vi "UI_Example.vi"() -> ()   [LabVIEW 2018]
uses:
  UI_Library/UI_Library.lvclass
  test/ClassData/ClassData.lvclass
  UI_Library.lvlib
  d44c3c8a-f4a9-44f0-87a1-e82cc9f3e378.vi
  bafeb2e0-969a-4f59-9125-878fceaa8550.vi
panel:
  in  "UI_Cluster":cluster{"Strg":string}
  out "Stopped":bool
  in  "Stop":bool
  out "NewVal":bool
  in  "UI_Strg":string
  in  "UI_Boolean":bool
  out "#el_queue":i32
  # "Example\nThis example highlights how the new library enables a fully decoupled architecture, allowing the Backend logic to operate independently and effortlessly from the UI layer.\nThanks to this library, UI interaction becomes cleaner, safer, and dramatically easier to maintain.\nSee Block Diagram Comment for more details!\n\nAnd the best part:\nThe library automatically manages all UI control references—zero boilerplate, zero coupling, maximum flexibility\nThe UI stays continuously updated by reference using a dedicated loop, ensuring smooth UI responsiveness without ever slowing down the Backend"
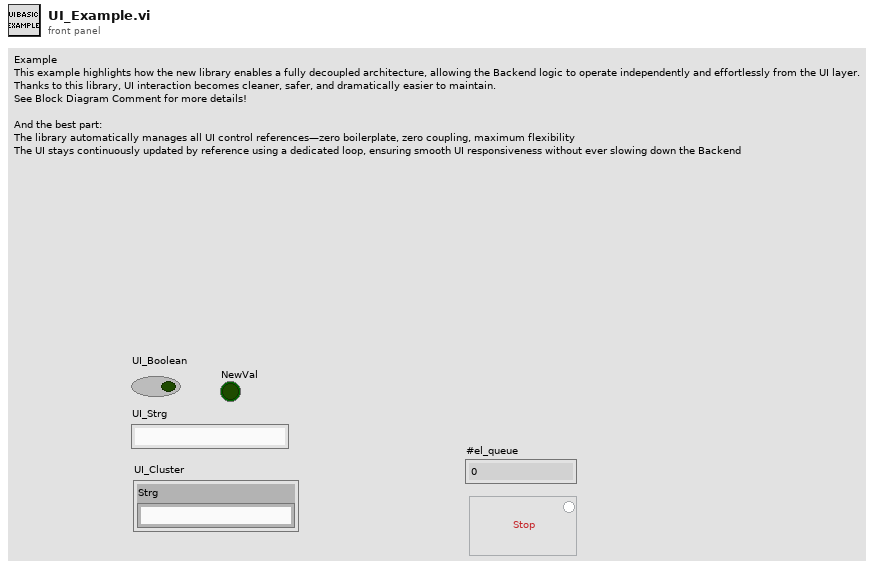
[diagram p1: front panel]
types:
  T1 = enum8{"Enabled", "Disabled", "Disabled and Grayed Out"}
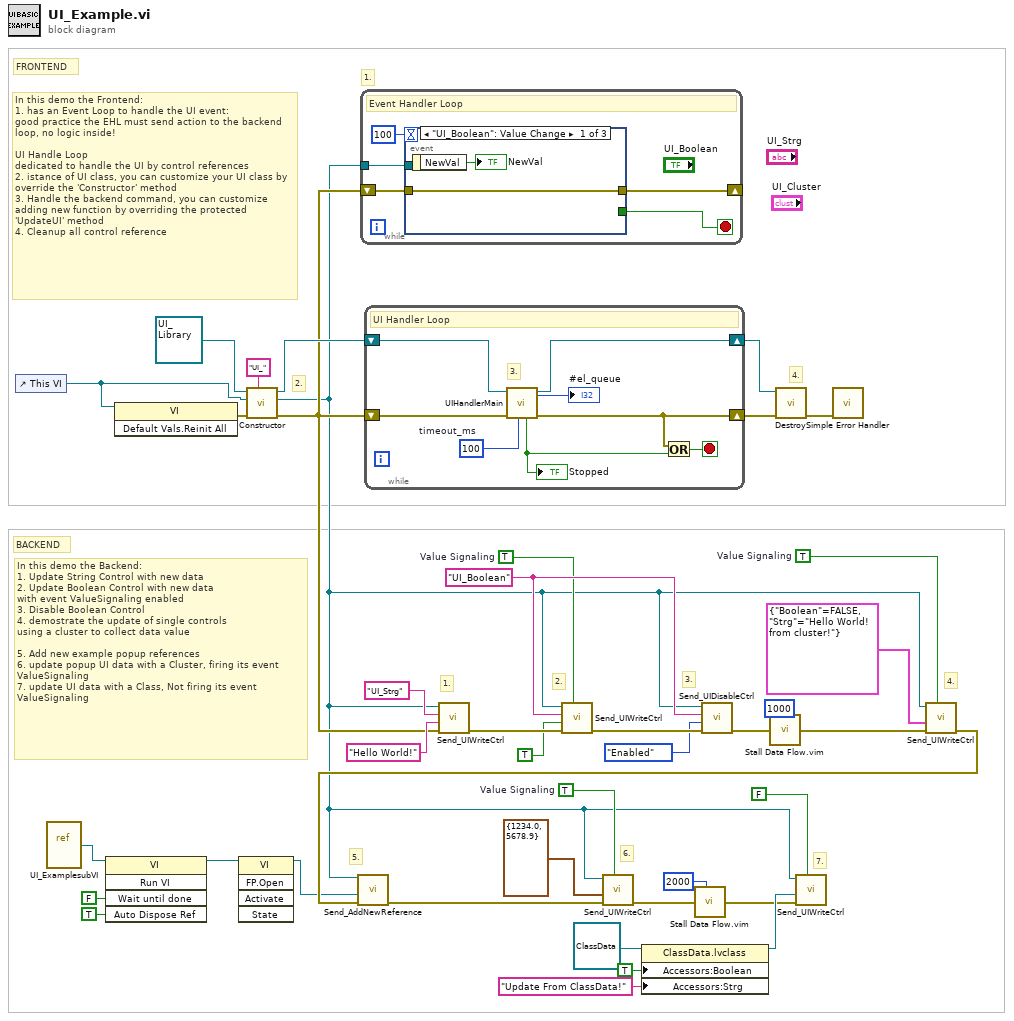
[diagram p0: block diagram]
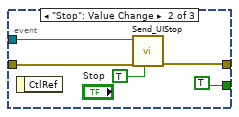
[diagram p2: hidden frame]
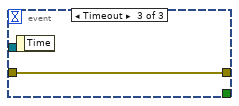
[diagram p3: hidden frame]
diagram:
  w16 = TRUE  # Value Signaling
  w21 = TRUE  # Value Signaling
  w24 = TRUE  # Value Signaling
  w26 = "UI_Boolean"
  # "7."
  # "6."
  # "5."
  # "4."
  # "2."
  # "1."
  # "In this demo the Frontend:\n1. has an Event Loop to handle the UI event: \ngood practice the EHL must send action to the backend loop, no logic inside!\n\nUI Handle Loop\ndedicated to handle the UI by control references\n2. istance of UI class, you can customize your UI class by override the 'Constructor' method\n3. Handle the backend command, you can customize adding new function by overriding the protected 'UpdateUI' method\n4. Cleanup all control reference"
  # "4."
  # "3."
  # "2."
  # "1."
  # "In this demo the Backend:\n1. Update String Control with new data\n2. Update Boolean Control with new data \nwith event ValueSignaling enabled\n3. Disable Boolean Control\n4. demostrate the update of single controls \nusing a cluster to collect data value\n\n5. Add new example popup references\n6. update popup UI data with a Cluster, firing its event ValueSignaling\n7. update UI data with a Class, Not firing its event ValueSignaling"
  # "BACKEND"
  # "FRONTEND"
  n1 = control-ref of="This VI"() -> (w29:refnum<vi>)
  n2 = vi-ref "UI_ExamplesubVI.vi"() -> (w14:refnum<vi>)
  n3 = invoke class="VI" method="Run VI"(reference=w14, "Wait until done"=FALSE ("Wait Until Done"), "Auto Dispose Ref"=TRUE ("Auto Dispose Reference")) -> (reference out=w11:refnum<vi>)  [unwired: 2 in, 4 out]
  n4 = invoke class="VI" method="Default Vals.Reinit All"(reference=w29) -> (error out=w28:errorcluster)  [unwired: 2 in, 2 out]
  n5 = invoke class="VI" method="FP.Open"(reference=w11) -> (reference out=w10:refnum<vi>)  [unwired: 4 in, 4 out]
  n6 = call-dynamic "Constructor.vi"("FP_Control_Flag"="UI_", "error in"=w28, "UI_Ref"=w29, "UI_Manager in"=refnum<class "UI_Library.lvclass"> refnum) -> ("error out"=w27:errorcluster, "UI_Queue"=w5:refnum<queue>, "UI_Manager out"=w37:refnum<class "UI_Library.lvclass">)  [unwired: 5 in]
  n7 = while {
    shift-right: [w44] -> _
    shift-left: w27 -> [w45]
    tunnel: w5 -> [w42]
    stop <- w41 stop-if-true
    # "Event Handler Loop"
    n8 = event shown="[0] \"UI_Boolean\": Value Change" {
      selector: _ -> [_ _ _]
      dyn-events: _ -> [_ _ _]
      timeout: 100 -> [_ _ _]
      tunnel: w45 -> [w47 w52 w53]
      tunnel: [w47 w51 w53] -> w44
      tunnel: w42 -> [_ w50 _]
      tunnel: [_ TRUE _] -> w41
      event "UI_Boolean": Value Change {
        n9 = event-data() -> ("NewVal"=→"NewVal":bool)  [unwired: 1 in]
      }
      event "Stop": Value Change {
        n10 = event-data() -> ()  [unwired: 1 in, 1 out]
        n11 = call "Send_UIStop.vi"("HighPriority (F)"=TRUE, "error in"=w52, "Queue in"=w50) -> ("error out"=w51:errorcluster)  [unwired: 8 in]
      }
      event Timeout {
        n12 = event-data() -> ()  [unwired: 1 in, 1 out]
      }
    }
  }
  n13 = while {
    shift-right: [w59] -> w39
    shift-left: w27 -> [w60]
    shift-right: [w57] -> w36
    shift-left: w37 -> [w58]
    stop <- w61 stop-if-true
    w56 = 100  # timeout_ms
    # "3."
    # "UI Handler Loop"
    n14 = call "UIHandlerMain.vi"("timeout_ms"=w56, "error in"=w60, "UI_Manager in"=w58) -> ("error out"=w59:errorcluster, "UI_Manager out"=w57:refnum<class "UI_Library.lvclass">, "CloseUILoop"=w54:bool, "#el_queue"=→"#el_queue":i32)  [unwired: 5 in]
    "Stopped" <- w54
    n15 = Or(x=w59, y=w54) -> (x .or. y?=w61:bool)
  }
  n16 = call "Send_UIWriteCtrl.vi"("error in"=w27, "Control Data"="Hello World!", "Control Label"="UI_Strg", "Queue in"=w5) -> ("error out"=w32:errorcluster)  [unwired: 7 in]
  n17 = call "Send_UIWriteCtrl.vi"("Value Signaling (F)"=w24, "error in"=w32, "Control Data"=TRUE, "Control Label"=w26, "Queue in"=w5) -> ("error out"=w31:errorcluster)  [unwired: 6 in]
  n18 = property class="ClassData.lvclass"(reference=refnum<class "ClassData.lvclass"> refnum ("ClassData.lvclass"), "Accessors:Boolean"=TRUE ("Boolean"), "Accessors:Strg"="Update From ClassData!" ("Strg")) -> (reference out=w6:refnum<class "ClassData.lvclass">)  [unwired: 1 in, 1 out]
  n19 = call "Send_UIDisableCtrl.vi"("error in"=w31, "Disabled"=T1."Enabled", "Control Label"=w26, "Queue in"=w5) -> ("error out"=w23:errorcluster)  [unwired: 7 in]
  n20 = call "Stall Data Flow.vim"("value in"=w23, "milliseconds to wait"=u32 1000) -> ("value out"=w20:errorcluster)  [unwired: 1 out]
  n21 = call-dynamic "Destroy.vi"("error in"=w39, "UI_Manager in"=w36) -> ("error out"=w38:errorcluster)  [unwired: 8 in, 1 out]
  n22 = call <vilib>:"Simple Error Handler.vi"("error in (no error)"=w38) -> ()  [unwired: 4 in, 5 out]
  n23 = call "Send_UIWriteCtrl.vi"("Value Signaling (F)"=w21, "error in"=w20, "Control Data"=cluster{"Boolean":bool, "Strg":string} {"Boolean"=FALSE, "Strg"="Hello World! from cluster!"}, "Queue in"=w5) -> ("error out"=w18:errorcluster)  [unwired: 7 in]
  n24 = call "Send_AddNewReference.vi"("error in"=w18, "NewRef"=w10, "Queue in"=w5) -> ("error out"=w17:errorcluster)  [unwired: 8 in]
  n25 = call "Send_UIWriteCtrl.vi"("Value Signaling (F)"=w16, "error in"=w17, "Control Data"=cluster{"Num1":dbl, "Num2":dbl} {"Num1"=1234.0, "Num2"=5678.9}, "Queue in"=w5) -> ("error out"=w3:errorcluster)  [unwired: 7 in]
  n26 = call "Stall Data Flow.vim"("value in"=w3, "milliseconds to wait"=u32 2000) -> ("value out"=w2:errorcluster)  [unwired: 1 out]
  n27 = call "Send_UIWriteCtrl.vi"("Value Signaling (F)"=FALSE, "error in"=w2, "Control Data"=w6, "Queue in"=w5) -> ()  [unwired: 7 in, 1 out]
